vi "test Acyclic Frames Section.vi"(8 "error in":errorcluster, 11 "TestCase in":refnum<class "Scripting.lvclass">) -> (0 "error out":errorcluster, 3 "TestCase out":refnum<class "Scripting.lvclass">)   [LabVIEW 2020, in "Scripting.lvclass"]
uses:
  Scripting.lvclass
  Scripting/AIM MIL-STD-1553 Scripting.lvlib
  <vilib>/addons/_JKI Toolkits/VI Tester/TestCase.llb/TestCase.lvclass
  Shared/Acyclic Frame Definition.ctl
  C:/dev/git/niveristand-custom-device-testing-tools/VeriStandScriptingTestCase/VeriStandScriptingTestCase.lvclass
  C:/Program Files (x86)/National Instruments/LabVIEW 2020/vi.lib/addons/_JKI Toolkits/VI Tester/TestCase.llb/TestCase.lvclass
  C:/dev/git/niveristand-aim-milStd1553-custom-device/Source/Custom Device Support/Tests/Unit/Scripting/Scripting.lvclass
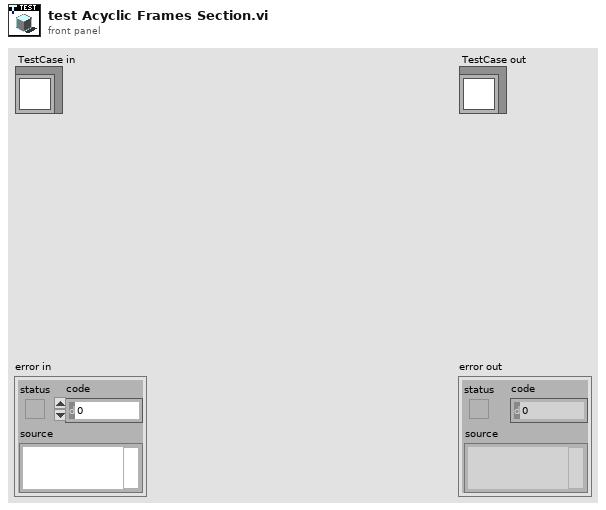
[diagram p1: front panel]
types:
  T1 = typedef "Acyclic Frame Definition.ctl" = cluster{"name":string, "messages":string[]}
  T2 = typedef "Custom Device API.lvlib/Custom Device Item Ref.ctl" = u64
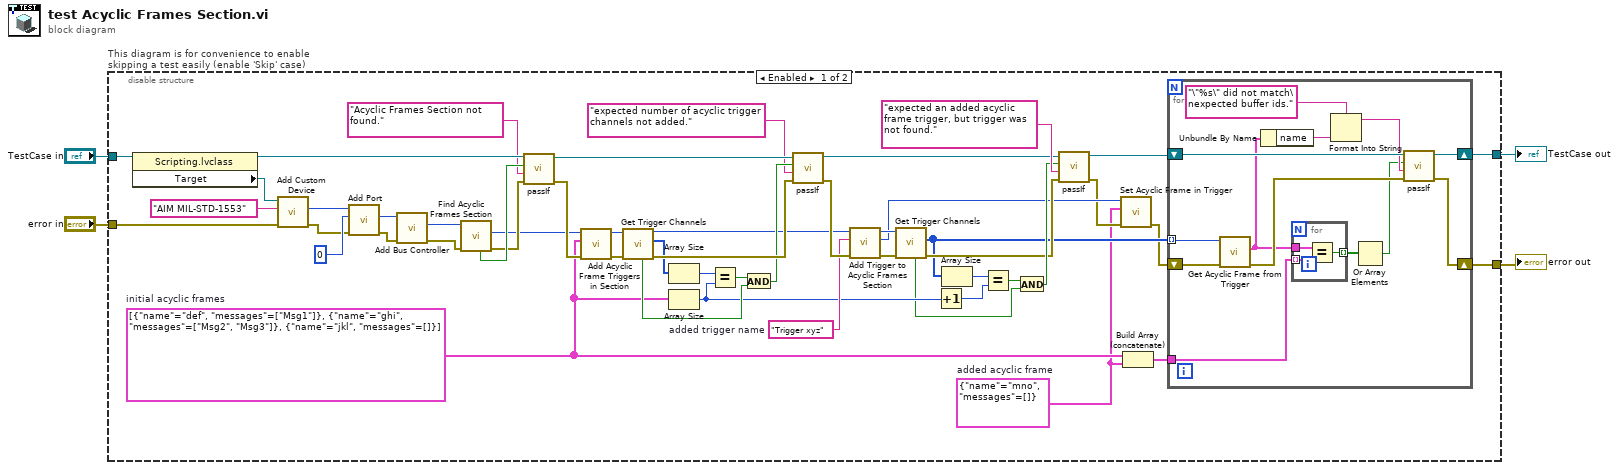
[diagram p0: block diagram]
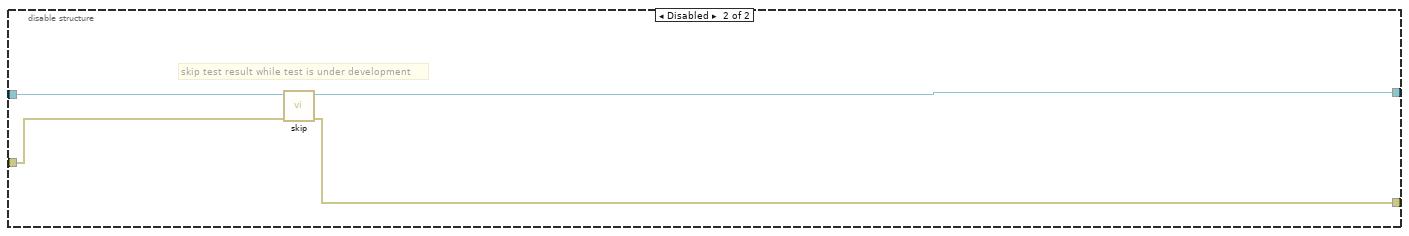
[diagram p2: hidden frame]
diagram:
  n1 = disable-structure "This diagram is for convenience to enable skipping a test easily (enable 'Skip' case)" shown="Enabled" {
    disable-tunnel: "TestCase in" -> [w53 w75]
    disable-tunnel: [w8 w73] -> w4
    disable-tunnel: [w7 w74] -> w2
    disable-tunnel: "error in" -> [w55 w72]
    frame Enabled {
      w5 = T1 {"name"="mno", "messages"=[]}  # added acyclic frame
      w6 = T1[] [{"name"="def", "messages"=["Msg1"]}, {"name"="ghi", "messages"=["Msg2", "Msg3"]}, {"name"="jkl", "messages"=[]}]  # initial acyclic frames
      w33 = "Trigger xyz"  # added trigger name
      n2 = property class="Scripting.lvclass"(reference=w53) -> (reference out=w40:refnum<class "Scripting.lvclass">, "Target"=w52:refnum<k24>)  [unwired: 1 in, 1 out]
      n3 = call "Add Custom Device.vi"("error in"=w55, "custom device name"="AIM MIL-STD-1553" ("name"), "target"=w52) -> ("error out"=w50:errorcluster, "custom device"=w49:T2)  [unwired: 6 in, 1 out]
      n4 = call "Add Port.vi"("error in"=w50, "port number"=u16 0, "custom device"=w49) -> ("error out"=w48:errorcluster, "port"=w47:T2)  [unwired: 6 in, 1 out]
      n5 = call "Add Bus Controller.vi"("error in"=w48, "port"=w47) -> ("error out"=w26:errorcluster, "bus controller"=w25:T2)  [unwired: 7 in, 1 out]
      n6 = call "Find Acyclic Frames Section.vi"("error in"=w26, "bus controller"=w25) -> ("error out"=w37:errorcluster, "acyclic frames section"=w21:T2, "found?"=w38:bool)  [unwired: 6 in, 1 out]
      n7 = call-dynamic "passIf.vi"("error in (no error)"=w37, "message (\"\")"="Acyclic Frames Section not found.", "pass"=w38, "TestCase in"=w40) -> ("error out"=w23:errorcluster, "TestCase out"=w39:refnum<class "Scripting.lvclass">)  [unwired: 6 in]
      n8 = call "Add Acyclic Frame Triggers in Section.vi"("error in"=w23, "acyclic frames"=w6, "acyclic frames section"=w21) -> ("error out"=w22:errorcluster, "acyclic frames section out"=w20:T2)  [unwired: 7 in]
      n9 = call "Get Trigger Channels.vi"("error in"=w22, "acyclic frames section"=w20) -> ("error out"=w46:errorcluster, "acyclic frame triggers"=w45:T2[], "acyclic frames section out"=w34:T2, "found?"=w42:bool)  [unwired: 6 in]
      n10 = Array Size(array=w45) -> (size(s)=w44:i32)
      n11 = Array Size(array=w6) -> (size(s)=w30:i32)
      n12 = Equal?(x=w44, y=w30) -> (x = y?=w43:bool)
      n13 = And(x=w43, y=w42) -> (x .and. y?=w41:bool)
      n14 = call-dynamic "passIf.vi"("error in (no error)"=w46, "message (\"\")"="expected number of acyclic trigger channels not added.", "pass"=w41, "TestCase in"=w39) -> ("error out"=w35:errorcluster, "TestCase out"=w18:refnum<class "Scripting.lvclass">)  [unwired: 6 in]
      n15 = call "Add Trigger to Acyclic Frames Section.vi"("error in"=w35, "trigger name"=w33, "acyclic frames section"=w34) -> ("error out"=w32:errorcluster, "acyclic frame trigger"=w14:T2, "acyclic frames section out"=w31:T2)  [unwired: 6 in]
      n16 = call "Get Trigger Channels.vi"("error in"=w32, "acyclic frames section"=w31) -> ("error out"=w15:errorcluster, "acyclic frame triggers"=w12:T2[], "found?"=w17:bool)  [unwired: 6 in, 1 out]
      n17 = Increment(x=w30) -> (x+1=w27:i32)
      n18 = Array Size(array=w12) -> (size(s)=w28:i32)
      n19 = Equal?(x=w28, y=w27) -> (x = y?=w29:bool)
      n20 = And(x=w29, y=w17) -> (x .and. y?=w16:bool)
      n21 = call-dynamic "passIf.vi"("error in (no error)"=w15, "message (\"\")"="expected an added acyclic frame trigger, but trigger was not found.", "pass"=w16, "TestCase in"=w18) -> ("error out"=w13:errorcluster, "TestCase out"=w10:refnum<class "Scripting.lvclass">)  [unwired: 6 in]
      n22 = call "Set Acyclic Frame in Trigger.vi"("error in"=w13, "acyclic frame"=w5, "acyclic frame trigger"=w14) -> ("error out"=w11:errorcluster)  [unwired: 7 in, 1 out]
      n23 = Build Array (concatenate)(w6, w5) -> (w9:T1[])
      n24 = for {
        tunnel: w12 -> [w68] mode=indexing
        tunnel: w9 -> [w58]
        shift-right: [w62] -> w7
        shift-left: w11 -> [w67]
        shift-right: [w61] -> w8
        shift-left: w10 -> [w66]
        n25 = call "Get Acyclic Frame from Trigger.vi"("error in"=w67, "acyclic frame trigger"=w68) -> ("error out"=w65:errorcluster, "acyclic frame out"=w60:T1)  [unwired: 6 in, 2 out]
        n26 = Unbundle By Name(w60) -> ("name"=w59:string)
        n27 = for {
          tunnel: w60 -> [w71]
          tunnel: w58 -> [w70] mode=indexing
          tunnel: [w69] -> w57 mode=indexing
          n28 = Equal?(x=w71, y=w70) -> (x = y?=w69:bool)
        }
        n29 = Format Into String(format string="\"%s\" did not match\nexpected buffer ids.", w59) -> (resulting string=w63:string)  [unwired: 2 in, 1 out]
        n30 = Or Array Elements(Boolean array=w57) -> (logical OR=w56:bool)
        n31 = call-dynamic "passIf.vi"("error in (no error)"=w65, "message (\"\")"=w63, "pass"=w56, "TestCase in"=w66) -> ("error out"=w62:errorcluster, "TestCase out"=w61:refnum<class "Scripting.lvclass">)  [unwired: 6 in]
      }
    }
    frame Disabled {
      # "skip test result while test is under development"
      n32 = call <vilib>:"skip.vi"("error in (no error)"=w72, "TestCase in"=w75) -> ("error out"=w74:errorcluster, "TestCase out"=w73:refnum<class "Scripting.lvclass">)  [unwired: 8 in]
    }
  }
  "error out" <- w2
  "TestCase out" <- w4
